vi "LabVIEW Code.vi"() -> ()   [LabVIEW 2013]
panel:
  in  "Tab Control":enum32{"Page 1", "Page 2"}(tab)
  out "Very Dry":bool
  out "Dry":bool
  out "Moist":bool
  out "Saturated":bool
  out "MEDIUM DANGER\n indicator":bool
  out "SAFE \nindicator":bool
  out "LOW WARNING  \n     indicator":bool
  out "HIGH DANGER\n indicator":bool
  out "CRITICAL":bool
  out "current time":timestamp format="%<%I:%M:%S %p\n%x>T"
  out "Node 1 Link Quality":sgl
  out "Node 2Link Quality":sgl
  out "air temprature":sgl(slide) scale=0.0..482.0
  out "soil temprature":sgl(slide) scale=0.0..482.0
  out "PMM SCALING CO":dbl(knob) scale=0.0..500.0
  out "heavy smoldring ambustion":bool
  out "light smoldring ambustion":bool
  out "CO2 Danger":bool
  in  "Stop Button":bool
  out "?":dbl(slide)
  out "CO2 PPM":dbl(knob) scale=0.0..10000.0
  out "Soil moiture sensor voltage":sgl(graph)
  out "MQ 7 voltage":sgl(graph)
  out "MQ 135 voltage":sgl(graph)
  out "date rv from py":string
  out "string rv in\n danger level loop":string
  out "resulting string sendingto python":string
  out "current time 2":timestamp
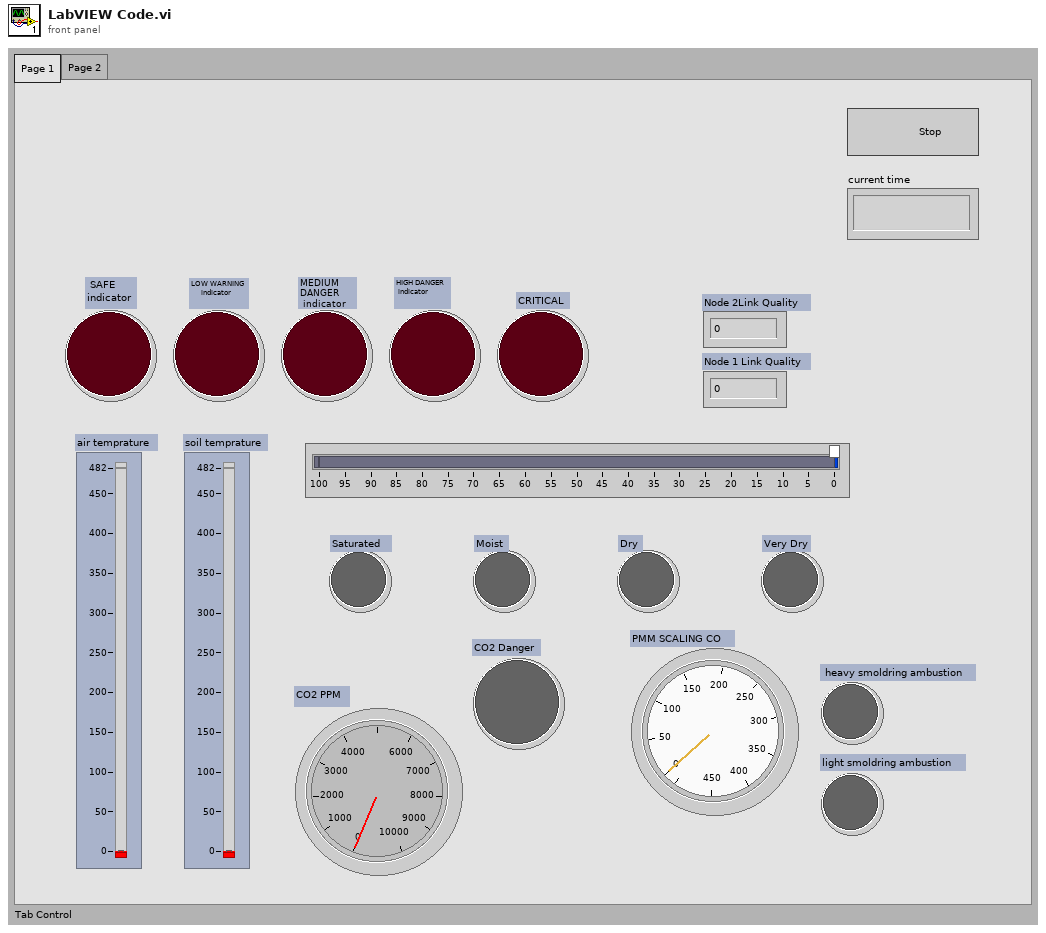
[diagram p1: front panel]
types:
  T1 = enum16{"open", "replace", "create", "open or create", "replace or create", "replace or create with confirmation"}
  T2 = enum16{"Standard", "Buffered", "CRLF", "Immediate"}
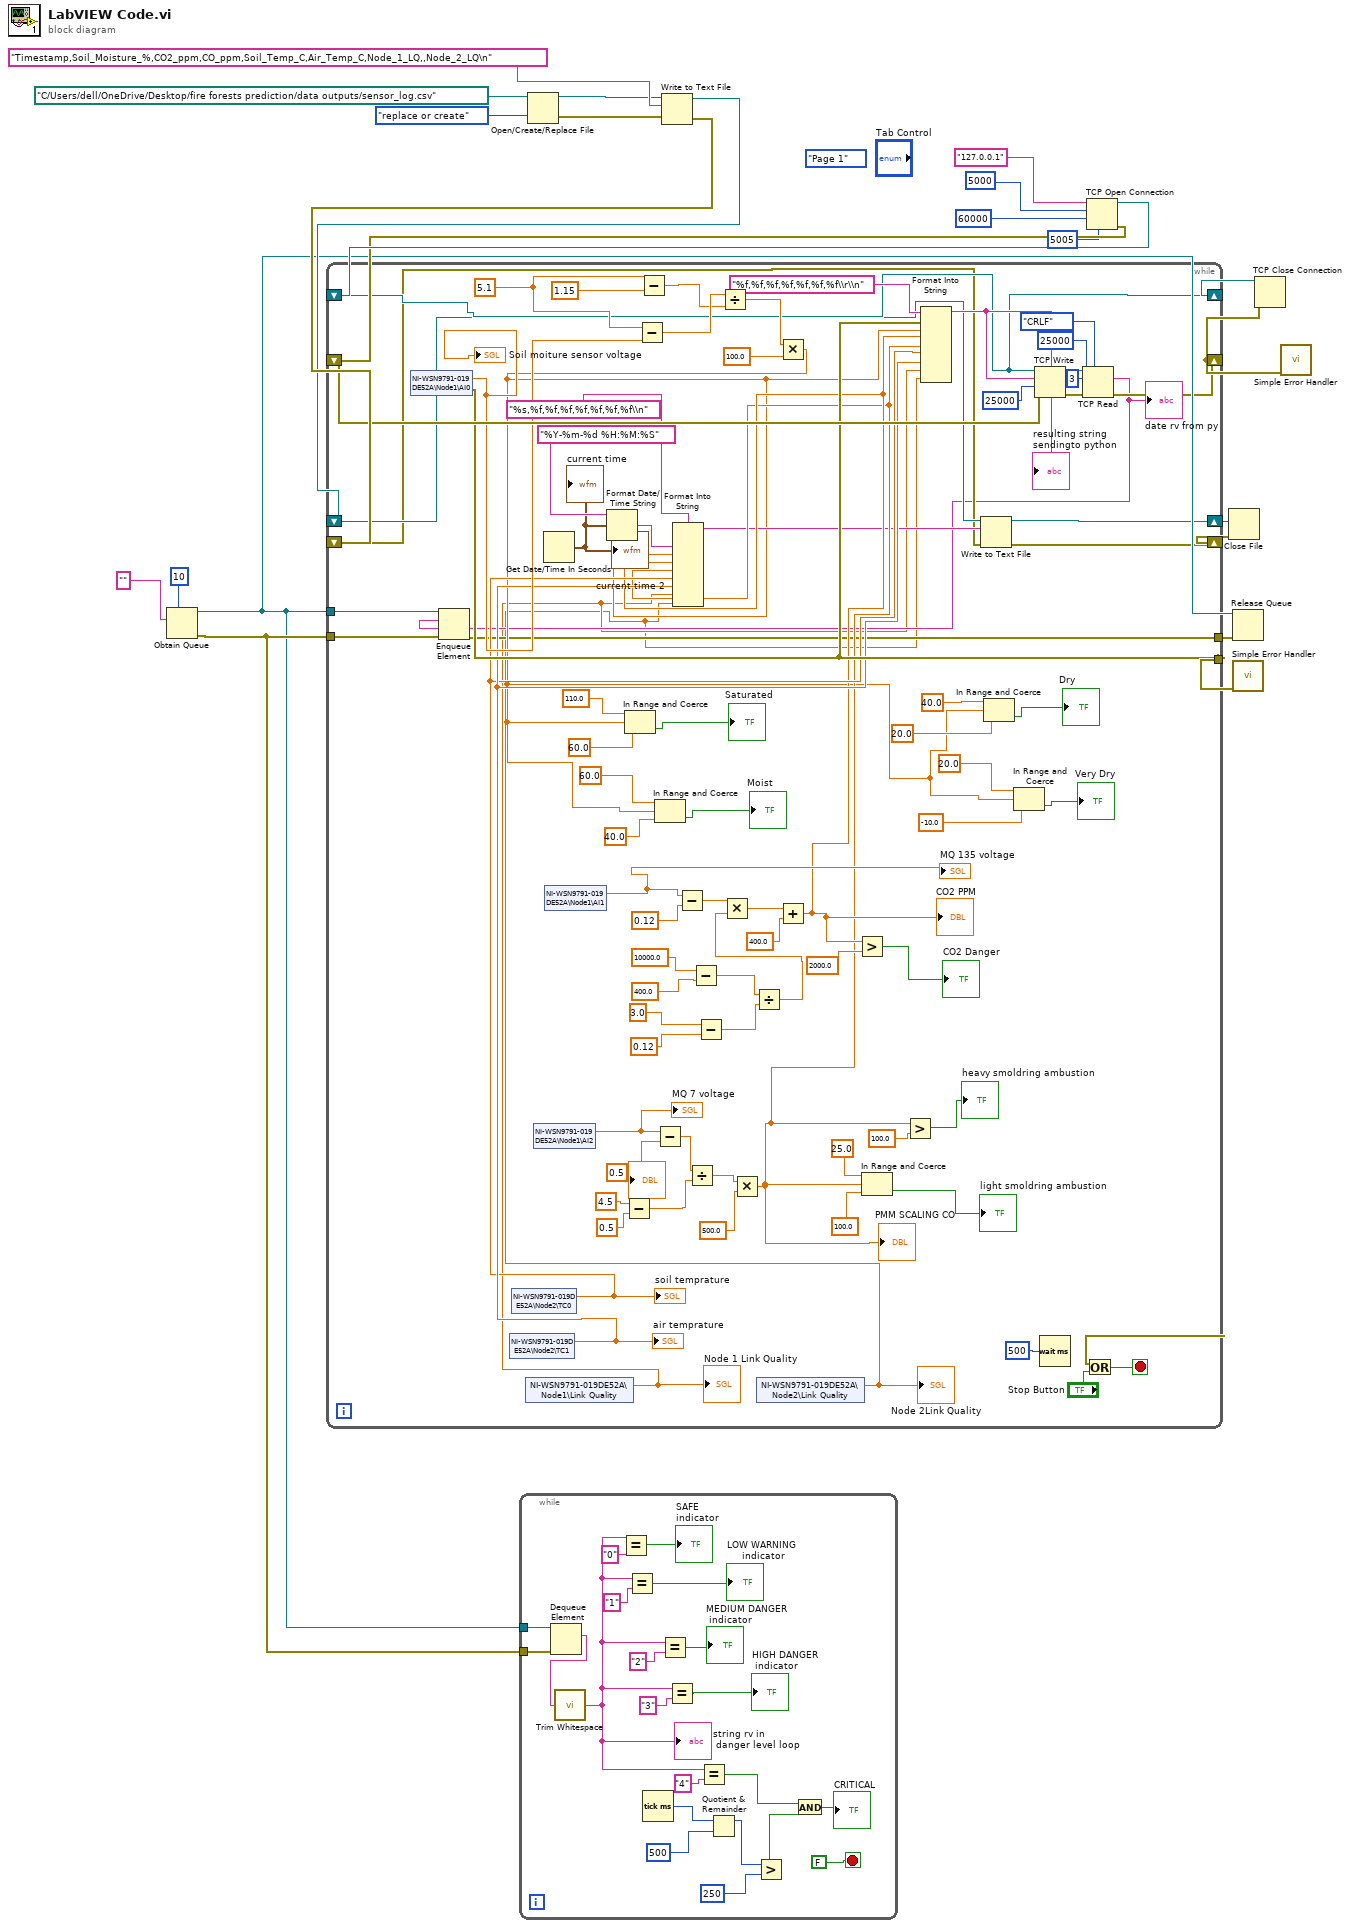
[diagram p0: block diagram]
diagram:
  (unwired) enum32{"Page 1", "Page 2"}."Page 1" ("Tab Control")
  n1 = Obtain Queue(max queue size (-1, unlimited)=10, element data type="") -> (queue out=w2:refnum<queue>, error out=w4:errorcluster)  [unwired: 3 in, 1 out]
  n2 = while {
    tunnel: w4 -> [w43]
    tunnel: w2 -> [w42]
    stop <- FALSE stop-if-true
    n3 = Dequeue Element(queue=w42, error in (no error)=w43) -> (element=w25:string)  [unwired: 1 in, 3 out]
    n4 = call <vilib>:"Trim Whitespace.vi"("string"=w25) -> ("trimmed string"=w24:string)  [unwired: 1 in]
    "string rv in\n danger level loop" <- w24
    n5 = Equal?(x=w24, y="0") -> (x = y?=→"SAFE \nindicator":bool)
    n6 = Equal?(x=w24, y="1") -> (x = y?=→"LOW WARNING  \n     indicator":bool)
    n7 = Tick Count (ms)() -> (millisecond timer value=w37:u32)
    n8 = Equal?(x=w24, y="2") -> (x = y?=→"MEDIUM DANGER\n indicator":bool)
    n9 = Equal?(x=w24, y="3") -> (x = y?=→"HIGH DANGER\n indicator":bool)
    n10 = Equal?(x=w24, y="4") -> (x = y?=w34:bool)
    n11 = Quotient & Remainder(x=w37, y=u32 500) -> (x-y*floor(x/y)=w31:u32)  [unwired: 1 out]
    n12 = Greater?(x=w31, y=u32 250) -> (0:w33:bool)
    n13 = And(x=w34, y=w33) -> (x .and. y?=→"CRITICAL":bool)
  }
  n14 = Open/Create/Replace File(file path (use dialog)=path "C:/Users/dell/OneDrive/Desktop/fire forests prediction/data outputs/sensor_log.csv", operation (0:open)=T1."replace or create") -> (refnum out=w14:refnum<file>, error out=w13:errorcluster)  [unwired: 4 in, 1 out]
  n15 = Write to Text File(file (use dialog)=w14, text="Timestamp,Soil_Moisture_%,CO2_ppm,CO_ppm,Soil_Temp_C,Air_Temp_C,Node_1_LQ,,Node_2_LQ\n", error in=w13) -> (refnum out=w8:refnum<file>, error out=w12:errorcluster)  [unwired: 1 in, 1 out]
  n16 = TCP Open Connection(address="127.0.0.1", remote port or service name=u16 5000, timeout ms (60000)=60000, local port=u16 5005 ("local port (0)")) -> (connection ID=w20:refnum<k5>, error out=w19:errorcluster)  [unwired: 1 in]
  n17 = while {
    tunnel: [w87] -> w23
    shift-right: [w59] -> w10
    shift-left: w12 -> [w61]
    shift-right: [w60] -> w11
    shift-left: w8 -> [w62]
    shift-right: [w101] -> w18
    shift-left: w20 -> [w101]
    shift-right: [w54] -> w6
    shift-left: w19 -> [w102]
    tunnel: w4 -> [w51]
    tunnel: [w50] -> w3
    tunnel: w2 -> [w49]
    stop <- w124 stop-if-true
    w122 = 5.1
    n18 = shared-variable "NI-WSN9791-019DE52A\\Node1\\AI0"() -> (w72:sgl, error out=w87:errorcluster)  [unwired: 1 in]
    "Soil moiture sensor voltage" <- w72
    n19 = shared-variable "NI-WSN9791-019DE52A\\Node2\\TC1"() -> (w68:sgl)  [unwired: 1 in, 1 out]
    "air temprature" <- w68
    n20 = shared-variable "NI-WSN9791-019DE52A\\Node2\\TC0"() -> (w67:sgl)  [unwired: 1 in, 1 out]
    "soil temprature" <- w67
    n21 = shared-variable "NI-WSN9791-019DE52A\\Node1\\Link Quality"() -> (w46:sgl)  [unwired: 1 in, 1 out]
    "Node 1 Link Quality" <- w46
    n22 = shared-variable "NI-WSN9791-019DE52A\\Node1\\AI2"() -> (w73:sgl)  [unwired: 1 in, 1 out]
    "MQ 7 voltage" <- w73
    n23 = Get Date/Time In Seconds() -> (seconds since 1Jan1904=w64:timestamp)
    "current time" <- w64
    "current time 2" <- w64
    n24 = shared-variable "NI-WSN9791-019DE52A\\Node1\\AI1"() -> (w74:sgl)  [unwired: 1 in, 1 out]
    "MQ 135 voltage" <- w74
    n25 = Format Date/Time String(time format string (%c)="%Y-%m-%d %H:%M:%S", seconds (now)=w64) -> (date/time string=w70:string)  [unwired: 1 in]
    n26 = Subtract(x=4.5, y=0.5) -> (x-y=w75:dbl)
    n27 = Subtract(x=w122, y=w72) -> (x-y=w121:dbl)
    n28 = Subtract(x=w122, y=1.15) -> (x-y=w120:dbl)
    n29 = Subtract(x=w73, y=0.5) -> (x-y=w85:dbl)
    n30 = Subtract(x=w74, y=0.12) -> (x-y=w99:dbl)
    n31 = Divide(x=w85, y=w75) -> (x/y=w84:dbl)
    n32 = Subtract(x=10000.0, y=400.0) -> (x-y=w92:dbl)
    n33 = Subtract(x=3.0, y=0.12) -> (x-y=w91:dbl)
    n34 = Divide(x=w121, y=w120) -> (x/y=w117:dbl)
    n35 = Multiply(x=w84, y=500.0) -> (x*y=w65:dbl)
    "PMM SCALING CO" <- w65
    n36 = Divide(x=w92, y=w91) -> (x/y=w90:dbl)
    n37 = Multiply(x=w99, y=w90) -> (x*y=w98:dbl)
    n38 = shared-variable "NI-WSN9791-019DE52A\\Node2\\Link Quality"() -> (w45:sgl)  [unwired: 1 in, 1 out]
    "Node 2Link Quality" <- w45
    n39 = Multiply(x=w117, y=100.0) -> (x*y=w57:dbl)
    n40 = In Range and Coerce(upper limit=110.0, x=w57, lower limit=60.0) -> (In Range?=→"Saturated":bool)  [unwired: 1 out]
    n41 = In Range and Coerce(upper limit=60.0, x=w57, lower limit=40.0) -> (In Range?=→"Moist":bool)  [unwired: 1 out]
    n42 = Add(x=w98, y=400.0) -> (x+y=w66:dbl)
    "CO2 PPM" <- w66
    n43 = Format Into String(format string="%s,%f,%f,%f,%f,%f,%f,%f\\n", w70, w57, w66, w65, w67, w68, w46, w45) -> (resulting string=w63:string)  [unwired: 2 in, 1 out]
    n44 = Greater?(x=w66, y=2000.0) -> (0:→"CO2 Danger":bool)
    n45 = In Range and Coerce(upper limit=25.0, x=w65, lower limit=100.0) -> (In Range?=→"light smoldring ambustion":bool)  [unwired: 1 out]
    n46 = Greater?(x=w65, y=100.0) -> (0:→"heavy smoldring ambustion":bool)
    n47 = Format Into String(format string="%f,%f,%f,%f,%f,%f,%f\\r\\n", error in=w87, w57, w66, w65, w67, w68, w46, w45) -> (resulting string=w103:string)  [unwired: 1 in, 1 out]
    "resulting string sendingto python" <- w103
    n48 = Write to Text File(file (use dialog)=w62, text=w63, error in=w61) -> (refnum out=w60:refnum<file>, error out=w59:errorcluster)  [unwired: 1 in, 1 out]
    n49 = In Range and Coerce(upper limit=40.0, x=w57, lower limit=20.0) -> (In Range?=→"Dry":bool)  [unwired: 1 out]
    n50 = In Range and Coerce(upper limit=20.0, x=w57, lower limit=-10.0) -> (In Range?=→"Very Dry":bool)  [unwired: 1 out]
    n51 = TCP Write(connection ID=w101, data in=w103, error in (no error)=w102, 9:25000 ("timeout ms (25000)")) -> (connection ID out=w56:refnum<k5>, error out=w55:errorcluster)  [unwired: 1 out]
    n52 = Wait (ms)(milliseconds to wait=u32 500) -> ()  [unwired: 1 out]
    n53 = TCP Read(connection ID=w56, bytes to read=3, error in (no error)=w55, 7:T2."CRLF" ("mode (standard)"), 9:25000 ("timeout ms (25000)")) -> (data out=w47:string, error out=w54:errorcluster)  [unwired: 1 out]
    "date rv from py" <- w47
    n54 = Enqueue Element(queue=w49, element=w47, error in (no error)=w51) -> (error out=w50:errorcluster)  [unwired: 1 in, 2 out]
    n55 = Or(x=w87, y="Stop Button") -> (x .or. y?=w124:bool)
  }
  n56 = Close File(refnum=w11, error in=w10) -> ()  [unwired: 2 out]
  n57 = Release Queue(queue=w2, error in (no error)=w3) -> ()  [unwired: 1 in, 3 out]
  n58 = call <vilib>:"Simple Error Handler.vi"("error in (no error)"=w23) -> ()  [unwired: 4 in, 5 out]
  n59 = TCP Close Connection(connection ID=w18, error in (no error)=w6) -> ()  [unwired: 1 in, 2 out]
  n60 = call <vilib>:"Simple Error Handler.vi"("error in (no error)"=w6) -> ()  [unwired: 4 in, 5 out]
